vi "oa_Check dr [OPS] (N Channels).vi"(8 "error in (no error)":errorcluster, 11 "resampled signal":cluster{"r0":dbl, "dr":dbl, "Y":dbl[]}[](array[cluster]) {"r0" format="%.2p"; "dr" format="%.2p"; "Y" format="%.2f"}) -> (0 "error out":errorcluster, 1 "parameter changed":bool, 3 "resampled signal out":cluster{"r0":dbl, "dr":dbl, "Y":dbl[]}[](array[cluster]))   [LabVIEW 2017, in "SoundVib_Resampling.lvlib"]
uses:
  <vilib>/addons/Sound and Vibration/Order Analysis/Resample Order Tracking/SoundVib_Resampling.lvlib
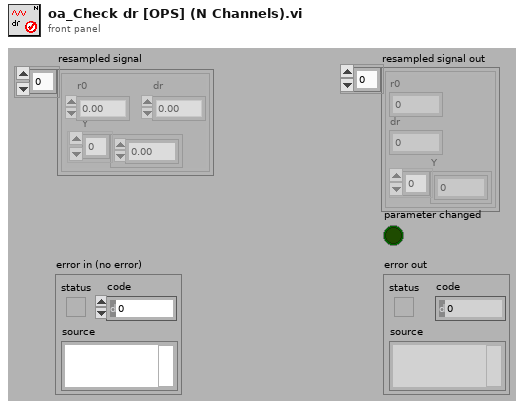
[diagram p1: front panel]
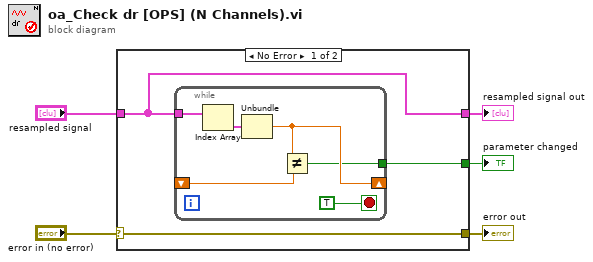
[diagram p0: block diagram]
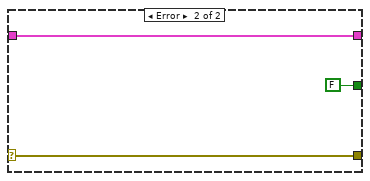
[diagram p2: hidden frame]
diagram:
  n1 = case shown="No Error" "error in (no error)" {
    selector: "error in (no error)" -> [w6 w17]
    tunnel: [w6 w17] -> w4
    tunnel: "resampled signal" -> [w8 w16]
    tunnel: [w8 w16] -> w2
    tunnel: [w7 FALSE] -> w1
    frame No Error {
      n2 = while {
        tunnel: w8 -> [w14]
        shift-right: [w11] -> _
        shift-left: _ -> [w12]
        tunnel: [w10] -> w7
        stop <- TRUE stop-if-true
        n3 = Index Array(array=w14) -> (element=w13:cluster{"r0":dbl, "dr":dbl, "Y":dbl[]})  [unwired: 1 in]
        n4 = Unbundle(w13) -> ("dr"=w11:dbl)  [unwired: 2 out]
        n5 = Not Equal?(x=w11, y=w12) -> (x != y?=w10:bool)
      }
    }
    frame Error {
    }
  }
  "error out" <- w4
  "resampled signal out" <- w2
  "parameter changed" <- w1
